vi "Mod_OFDM_Initialization.vi"(11 "error in (no error)":errorcluster) -> (4 "Configuration out":variant=variant("Data Source Pool "=variant(cluster{"mode (PN)":enum16{"PN", "pattern", "user"}, "PN sequence order (9)":i32, "base bit pattern (00001111)":enum16{"0", "1", "01", "0011", "00001111"}, "User base bit pattern":i8[]}[] [{"mode (PN)"=enum."PN", "PN sequence order (9)"=9, "base bit pattern (00001111)"=enum."00001111", "User base bit pattern"=[]}, {"mode (PN)"=enum."PN", "PN sequence order (9)"=9, "base bit pattern (00001111)"=enum."00001111", "User base bit pattern"=[]}, {"mode (PN)"=enum."PN", "PN sequence order (9)"=9, "base bit pattern (00001111)"=enum."00001111", "User base bit pattern"=[]}, {"mode (PN)"=enum."user", "PN sequence order (9)"=9, "base bit pattern (00001111)"=enum."00001111", "User base bit pattern"=[]}]), "FRAME Table"=variant(string[][] []), "Modulator Source Pool "=variant(cluster{"M-QAM":enum16{"4", "16", "64", "256", "1024"}, "M-PSK":enum16{"2", "4", "8", "16", "32", "64", "128", "256"}, "Type of Modulation":enum16{"PSK", "QAM"}, "PSK":cluster{"differential PSK":enum16{"disable", "enable"}, "PSK type":enum16{"normal", "shifted", "offset"}}}[] [{"M-QAM"=enum."4", "M-PSK"=enum."2", "Type of Modulation"=enum."PSK", "PSK"={"differential PSK"=enum."disable", "PSK type"=enum."normal"}}, {"M-QAM"=enum."4", "M-PSK"=enum."2", "Type of Modulation"=enum."PSK", "PSK"={"differential PSK"=enum."disable", "PSK type"=enum."normal"}}, {"M-QAM"=enum."4", "M-PSK"=enum."2", "Type of Modulation"=enum."PSK", "PSK"={"differential PSK"=enum."disable", "PSK type"=enum."normal"}}, {"M-QAM"=enum."4", "M-PSK"=enum."2", "Type of Modulation"=enum."PSK", "PSK"={"differential PSK"=enum."disable", "PSK type"=enum."normal"}}]), "OFDM Frame"=variant(cluster{"Symbol Name":string, "# of Symbols":i32}[] []), "OFDM SYMBOL POOL"=variant(string[] []), "Pulse Shaping"=variant(cluster{"System Filter":cluster{"TX Filter":enum16{"none", "Raised Cosine", "Root Raised Cos"}, "Alpha":dbl, "filter length":i32}, "Modulation system parameters":cluster{"samples per symbol (16)":i32}, "symbol rate (Hz)":dbl} {"System Filter"={"TX Filter"=enum."none", "Alpha"=0.0, "filter length"=0}, "Modulation system parameters"={"samples per symbol (16)"=0}, "symbol rate (Hz)"=0.0}), "Sub Carrier Selection"=variant(cluster{"Sub Carrier Selection":cluster{"Sub Carrier":bool, "Data Source":u16, "Modulator":u16}[], "OFDM Parameters":cluster{"# of Sub Carrier":i32, "Length Of Cylic Prefix":i32}} {"Sub Carrier Selection"=[{"Sub Carrier"=TRUE, "Data Source"=0, "Modulator"=0}, {"Sub Carrier"=TRUE, "Data Source"=0, "Modulator"=0}, {"Sub Carrier"=TRUE, "Data Source"=0, "Modulator"=0}, {"Sub Carrier"=TRUE, "Data Source"=0, "Modulator"=0}, {"Sub Carrier"=TRUE, "Data Source"=0, "Modulator"=0}, {"Sub Carrier"=TRUE, "Data Source"=0, "Modulator"=0}], "OFDM Parameters"={"# of Sub Carrier"=64, "Length Of Cylic Prefix"=16}}), "Symbol Table"=variant(string[][] [])), 15 "error out":errorcluster)   [LabVIEW 2010]
doc: "The VI initializes the configuration variant and sets the default values of the attribute like, pool of data sources, pool of modulator sources and pulse shaping parameters. These default values can be edited by changing the default values of the input controls."
uses:
  Controls(Type_DEf)/Attribute Names.ctl
  Controls(Type_DEf)/Pool of Data Source Control.ctl
  Controls(Type_DEf)/Pool of Modulator Control.ctl
  Controls(Type_DEf)/Configure Pulse Shaping.ctl
panel:
  in  "Pulse Shaping":T1={"System Filter"={"TX Filter"=enum."Root Raised Cos", "Alpha"=0.5, "filter length"=8}, "Modulation system parameters"={"samples per symbol (16)"=16}, "symbol rate (Hz)"=100000.0} {"symbol rate (Hz)" min=1.0 step=1.0 format="%.2p"; "Modulation system parameters"."samples per symbol (16)" step=2; "System Filter"."Alpha" min=0.0 max=1.0 step=0.05 format="%.2f"}
  in  "Sub Carrier Selection":T2={"Sub Carrier Selection"=array[10000 elements], "OFDM Parameters"={"# of Sub Carrier"=64, "Length Of Cylic Prefix"=16}}
  in  "Pool of Modulators":T3=[{"M-QAM"=enum."4", "M-PSK"=enum."2", "Type of Modulation"=enum."PSK", " PSK"={"differential PSK"=enum."disable", "PSK type"=enum."normal"}}, {"M-QAM"=enum."4", "M-PSK"=enum."2", "Type of Modulation"=enum."PSK", " PSK"={"differential PSK"=enum."disable", "PSK type"=enum."normal"}}, {"M-QAM"=enum."4", "M-PSK"=enum."2", "Type of Modulation"=enum."PSK", " PSK"={"differential PSK"=enum."disable", "PSK type"=enum."normal"}}, {"M-QAM"=enum."4", "M-PSK"=enum."2", "Type of Modulation"=enum."PSK", " PSK"={"differential PSK"=enum."disable", "PSK type"=enum."normal"}}]
  in  "Pool of Data Sources":T4=[{"mode (PN)"=enum."PN", "PN sequence order (9)"=9, "Invert Output Bits"=enum."No", "Register Initial State "=3602873842, "User base bit pattern"=[], "base bit pattern (00001111)"=enum."00001111", "Reset to Initial State"=enum."Every OFDM Frame"}, {"mode (PN)"=enum."PN", "PN sequence order (9)"=9, "Invert Output Bits"=enum."No", "Register Initial State "=3602873842, "User base bit pattern"=[], "base bit pattern (00001111)"=enum."00001111", "Reset to Initial State"=enum."Every OFDM Frame"}, {"mode (PN)"=enum."PN", "PN sequence order (9)"=9, "Invert Output Bits"=enum."No", "Register Initial State "=3602873842, "User base bit pattern"=[], "base bit pattern (00001111)"=enum."00001111", "Reset to Initial State"=enum."Every OFDM Frame"}, {"mode (PN)"=enum."PN", "PN sequence order (9)"=9, "Invert Output Bits"=enum."No", "Register Initial State "=3602873842, "User base bit pattern"=[], "base bit pattern (00001111)"=enum."00001111", "Reset to Initial State"=enum."Every OFDM Frame"}] {"Register Initial State" format="%08x"}
  in  "Atribute Names":T5={"Data Source Pool"="Data Source ", "Modulator Source Pool"="Modulator Source Pool ", "OFDM SYMBOL POOL"="OFDM SYMBOL POOL", "Symbol Table"="Symbol Table", "Sub Carrier Selection"="Sub Carrier Selection", "OFDM Frame"="OFDM Frame", "FRAME Table"="FRAME Table", "Pulse Shaping"="Pulse Shaping"}
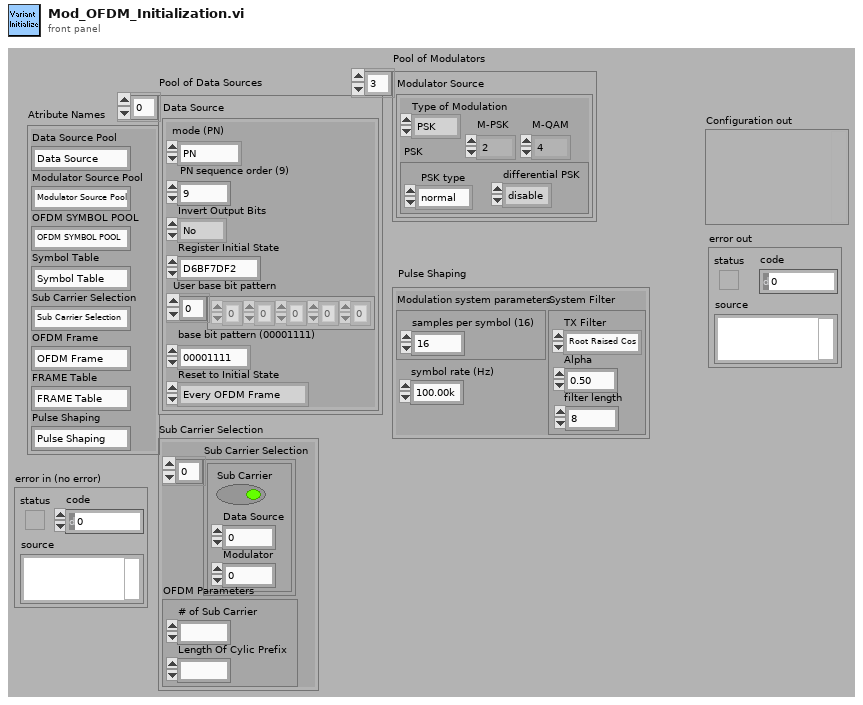
[diagram p1: front panel]
types:
  T1 = typedef "Configure Pulse Shaping.ctl" = cluster{"System Filter":cluster{"TX Filter":enum16{"none", "Raised Cosine", "Root Raised Cos"}, "Alpha":dbl, "filter length":i32}, "Modulation system parameters":cluster{"samples per symbol (16)":u32}, "symbol rate (Hz)":dbl}
  T2 = cluster{"Sub Carrier Selection":cluster{"Sub Carrier":bool, "Data Source":u16, "Modulator":u16}[], "OFDM Parameters":cluster{"# of Sub Carrier":i32, "Length Of Cylic Prefix":i32}}
  T3 = typedef "Pool of Modulator Control.ctl" = cluster{"M-QAM":enum16{"4", "16", "64", "256"}, "M-PSK":enum16{"2", "4", "8", "16", "32", "64", "128", "256"}, "Type of Modulation":enum16{"PSK", "QAM"}, " PSK":cluster{"differential PSK":enum16{"disable", "enable"}, "PSK type":enum16{"normal", "shifted", "offset"}}}[]
  T4 = typedef "Pool of Data Source Control.ctl" = cluster{"mode (PN)":enum16{"PN", "pattern", "user"}, "PN sequence order (9)":i32, "Invert Output Bits":enum16{"No", "Yes"}, "Register Initial State ":u32, "User base bit pattern":i8[], "base bit pattern (00001111)":enum16{"0", "1", "01", "0011", "00001111"}, "Reset to Initial State":enum16{"Every OFDM Frame", "Every OFDM Symbol", "Every Sub Carrier"}}[]
  T5 = typedef "Attribute Names.ctl" = cluster{"Data Source Pool":string, "Modulator Source Pool":string, "OFDM SYMBOL POOL":string, "Symbol Table":string, "Sub Carrier Selection":string, "OFDM Frame":string, "FRAME Table":string, "Pulse Shaping":string}
  T6 = cluster{"Symbol Name":string, "# of Symbols":i32}[]
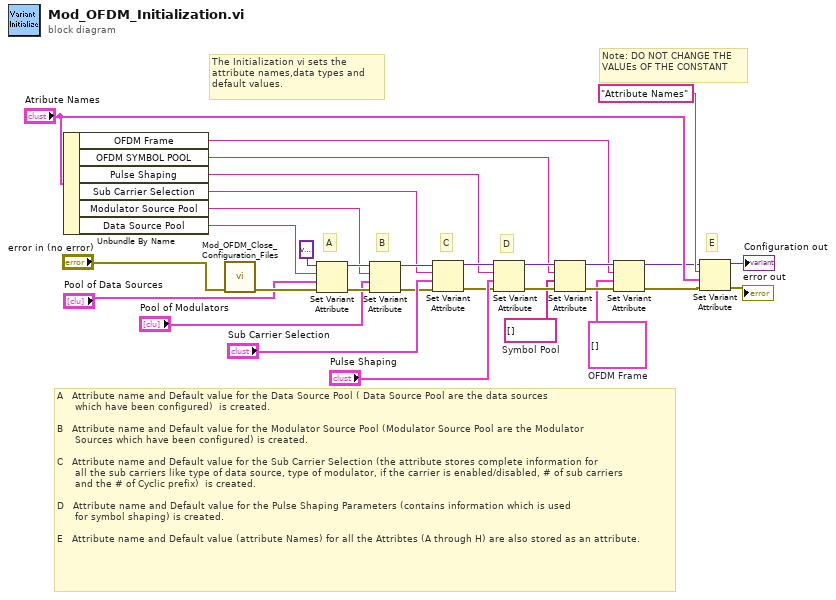
[diagram p0: block diagram]
diagram:
  w1 = string[] []  # Symbol Pool
  w2 = T6 []  # OFDM Frame
  # "A   Attribute name and Default value for the Data Source Pool ( Data Source Pool are the data sources \n      which have been configured)  is created.\n\nB   Attribute name and Default value for the Modulator Source Pool (Modulator Source Pool are the Modulator\n      Sources which have been configured) is created. \n\nC   Attribute name and Default value for the Sub Carrier Selection (the attribute stores complete information for \n      all the sub carriers like type of data source, type of modulator, if the carrier is enabled/disabled, # of sub carriers\n      and the # of Cyclic prefix)  is created.\n\nD   Attribute name and Default value for the Pulse Shaping Parameters (contains information which is used \n      for symbol shaping) is created.\n\nE   Attribute name and Default value (attribute Names) for all the Attribtes (A through H) are also stored as an attribute."
  # "E"
  # "D"
  # "C"
  # "A"
  # "B"
  # "The Initialization vi sets the attribute names,data types and default values."
  # "Note: DO NOT CHANGE THE VALUEs OF THE CONSTANT"
  n1 = Unbundle By Name("Atribute Names") -> ("OFDM Frame"=w3:string, "OFDM SYMBOL POOL"=w4:string, "Pulse Shaping"=w11:string, "Sub Carrier Selection"=w12:string, "Modulator Source Pool"=w28:string, "Data Source Pool"=w29:string)
  n2 = call "Mod_OFDM_Close_Configuration_Files.vi"("error in (no error)"="error in (no error)") -> ("error out"=w23:errorcluster)  [unwired: 14 in]
  n3 = Set Variant Attribute(Variant=variant, name=w29, value="Pool of Data Sources", error in=w23) -> (Variant out=w31:variant, error out=w30:errorcluster)  [unwired: 1 out]
  n4 = Set Variant Attribute(Variant=w31, name=w28, value="Pool of Modulators", error in=w30) -> (Variant out=w16:variant, error out=w15:errorcluster)  [unwired: 1 out]
  n5 = Set Variant Attribute(Variant=w16, name=w12, value="Sub Carrier Selection", error in=w15) -> (Variant out=w14:variant, error out=w13:errorcluster)  [unwired: 1 out]
  n6 = Set Variant Attribute(Variant=w14, name=w11, value="Pulse Shaping", error in=w13) -> (Variant out=w10:variant, error out=w7:errorcluster)  [unwired: 1 out]
  n7 = Set Variant Attribute(Variant=w10, name=w4, value=w1, error in=w7) -> (Variant out=w9:variant, error out=w6:errorcluster)  [unwired: 1 out]
  n8 = Set Variant Attribute(Variant=w9, name=w3, value=w2, error in=w6) -> (Variant out=w8:variant, error out=w5:errorcluster)  [unwired: 1 out]
  n9 = Set Variant Attribute(Variant=w8, name="Attribute Names", value="Atribute Names", error in=w5) -> (Variant out=→"Configuration out":variant, error out=→"error out":errorcluster)  [unwired: 1 out]
